vi "Unit Test Suite - JSON Schema Generator.vi"   [LabVIEW 2023, in "JSON Schema Generator.lvlib"]
uses:
  JSON Schema Generator.lvlib
  <vilib>/addons/_JKI Toolkits/Caraya/classes/Test Suite/Define Test Suite (Default).vi
  <vilib>/addons/_JKI Toolkits/Caraya/classes/Test Suite/Test Suite.lvclass
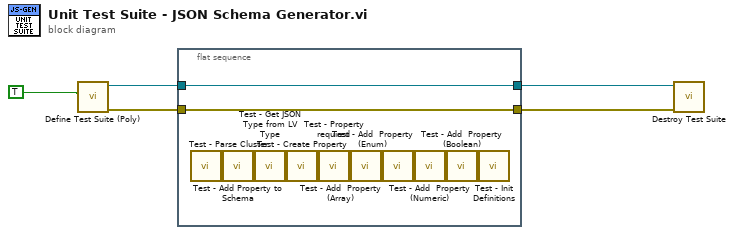
[diagram p0: block diagram]
diagram:
  n1 = call-poly <vilib>:"Define Test Suite (Poly).vi"("Interactive"=TRUE) -> ("error out"=w2:errorcluster, "Test Suite"=w4:refnum<class "Test Suite.lvclass">)  [unwired: 8 in, 1 out]
  n2 = flat-sequence {
    tunnel: [w7] -> w5
    tunnel: w4 -> [w7]
    tunnel: [w6] -> w3
    tunnel: w2 -> [w6]
    frame #0 {
      n3 = call "Test - Parse Cluster.vi"() -> ()  [unwired: 12 in]
      n4 = call "Test - Add Property to Schema.vi"() -> ()  [unwired: 12 in]
      n5 = call "Test - Get JSON Type from LV Type.vi"() -> ()  [unwired: 12 in]
      n6 = call "Test - Create Property.vi"() -> ()  [unwired: 12 in]
      n7 = call "Test - Property required.vi"() -> ()  [unwired: 12 in]
      n8 = call "Test - Add  Property (Array).vi"() -> ()  [unwired: 12 in]
      n9 = call "Test - Add  Property (Enum).vi"() -> ()  [unwired: 12 in]
      n10 = call "Test - Add  Property (Numeric).vi"() -> ()  [unwired: 12 in]
      n11 = call "Test - Add  Property (Boolean).vi"() -> ()  [unwired: 12 in]
      n12 = call "Test - Init Definitions.vi"() -> ()  [unwired: 12 in]
    }
  }
  n13 = call-dynamic "Destroy Test Suite.vi"("error in (no error)"=w3, "Test Suite in"=w5) -> ()  [unwired: 8 in, 2 out]
